vi "Configure Acquisition.vi"(0 "VISA resource name":refnum<visa-resource-name>, 1 "Enable Analog Averaging (Disable)":bool, 2 "Number Of Averages (8)":i32=8, 5 "Acquisition Type (0: Normal)":u16(ring) items=["Normal", "Peak Detect", "High Resolution"], 7 "Sampling Mode  (0: Real Time)":u16(ring) items=["Real Time", "Equivalent Time", "Segment"], 9 "Interpolation (0:No Interpolation)":u16(ring) items=["No Interpolation", "sin(x)/x"], 11 "error in (no error)":errorcluster, 12 "Segment Count (256)":i32=256) -> (4 "VISA resource name out":refnum<visa-resource-name>, 15 "error out":errorcluster)   [LabVIEW 2012, in "Agilent 8000 Series.lvlib"]
doc: "Configures how the oscilloscope acquires data and fills the waveform record."
uses:
  Agilent 8000 Series.lvlib
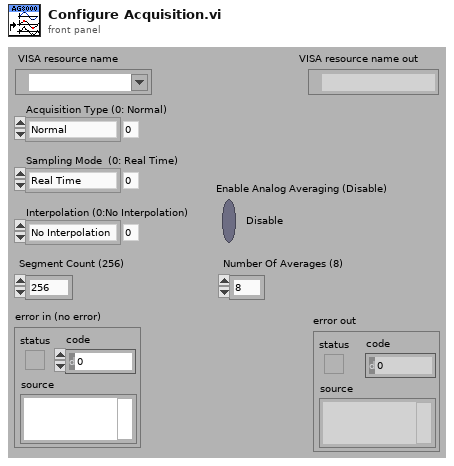
[diagram p1: front panel]
types:
  T1 = enum16{"Real Time", "Peak Detect", "High Resolution"}
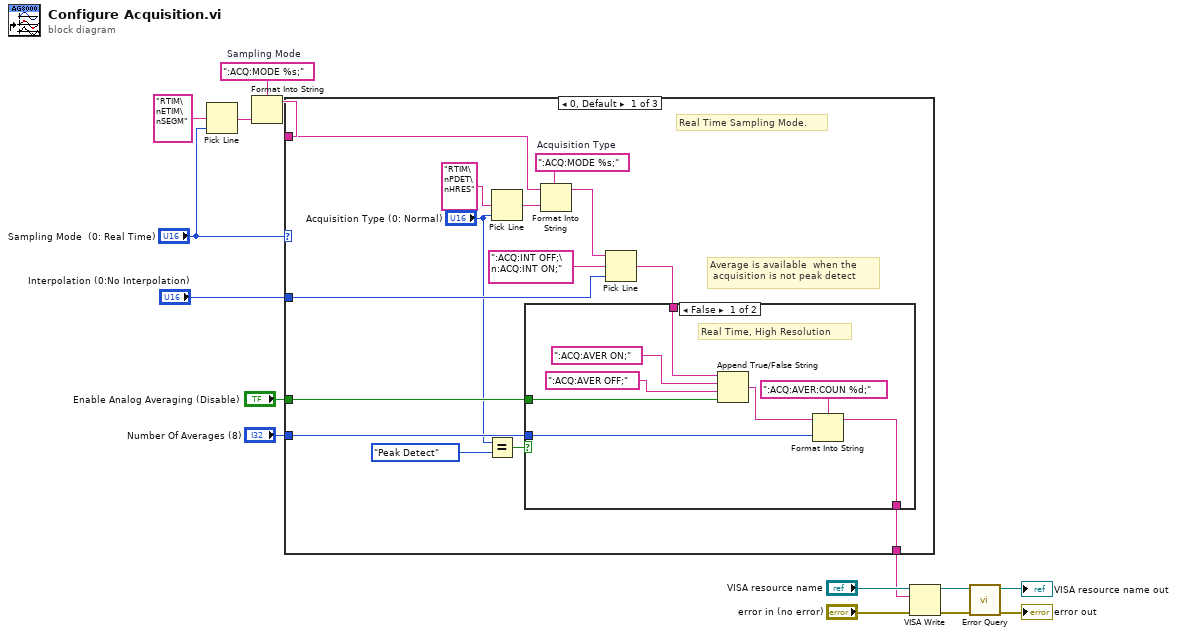
[diagram p0: block diagram]
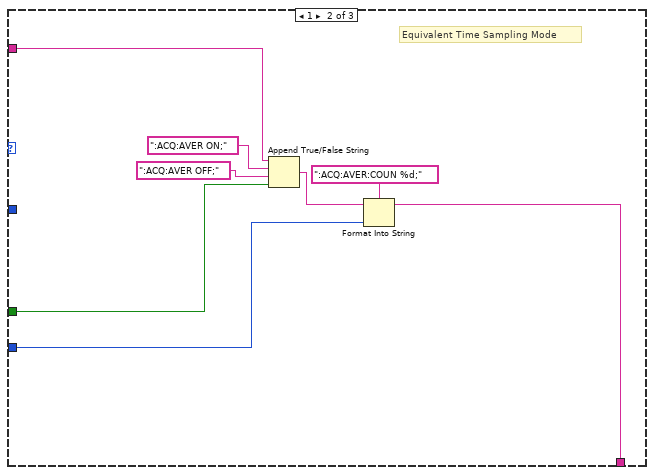
[diagram p3: hidden frame]
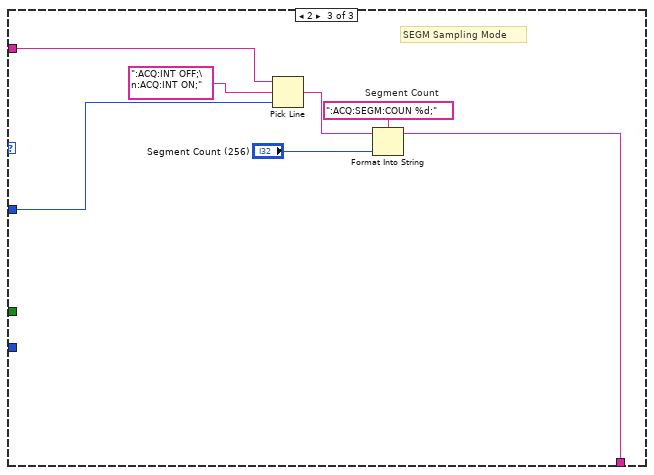
[diagram p4: hidden frame]
diagram:
  w8 = ":ACQ:MODE %s;"  # Sampling Mode
  n1 = Pick Line(multi-line string="RTIM\nETIM\nSEGM", line index="Sampling Mode  (0: Real Time)") -> (output string=w9:string)  [unwired: 1 in]
  n2 = Format Into String(format string=w8, w9) -> (resulting string=w6:string)  [unwired: 2 in, 1 out]
  n3 = case shown="0, Default" "Sampling Mode  (0: Real Time)" {
    tunnel: w6 -> [w16 w45 w52]
    tunnel: "Interpolation (0:No Interpolation)" -> [w28 _ w51]
    tunnel: "Enable Analog Averaging (Disable)" -> [w27 w46 _]
    tunnel: "Number Of Averages (8)" -> [w26 w42 _]
    tunnel: [w24 w39 w47] -> w2
    frame 0, Default {
      w23 = ":ACQ:MODE %s;"  # Acquisition Type
      # "Average is available  when the\n acquisition is not peak detect"
      # "Real Time Sampling Mode."
      n4 = Equal?(x="Acquisition Type (0: Normal)", y=T1."Peak Detect") -> (x = y?=w17:bool)
      n5 = Pick Line(multi-line string="RTIM\nPDET\nHRES", line index="Acquisition Type (0: Normal)") -> (output string=w22:string)  [unwired: 1 in]
      n6 = Format Into String(format string=w23, initial string=w16, w22) -> (resulting string=w20:string)  [unwired: 1 in, 1 out]
      n7 = Pick Line(string ("")=w20, multi-line string=":ACQ:INT OFF;\n:ACQ:INT ON;", line index=w28) -> (output string=w25:string)
      n8 = case shown="False" w17 {
        tunnel: w27 -> [w33 _]
        tunnel: w26 -> [w32 _]
        tunnel: w25 -> [w31 w38]
        tunnel: [w30 w38] -> w24
        frame False {
          # "Real Time, High Resolution"
          n9 = Append True/False String(1:w33, 2:":ACQ:AVER OFF;" ("false string"), 3:":ACQ:AVER ON;" ("true string"), 4:w31) -> (0:w37:string)
          n10 = Format Into String(format string=":ACQ:AVER:COUN %d;", initial string=w37, w32) -> (resulting string=w30:string)  [unwired: 1 in, 1 out]
        }
        frame True {
          # "Peak Detect"
        }
      }
    }
    frame 1 {
      # "Equivalent Time Sampling Mode"
      n11 = Append True/False String(1:w46, 2:":ACQ:AVER OFF;" ("false string"), 3:":ACQ:AVER ON;" ("true string"), 4:w45) -> (0:w40:string)
      n12 = Format Into String(format string=":ACQ:AVER:COUN %d;", initial string=w40, w42) -> (resulting string=w39:string)  [unwired: 1 in, 1 out]
    }
    frame 2 {
      w48 = ":ACQ:SEGM:COUN %d;"  # Segment Count
      # "SEGM Sampling Mode"
      n13 = Pick Line(string ("")=w52, multi-line string=":ACQ:INT OFF;\n:ACQ:INT ON;", line index=w51) -> (output string=w49:string)
      n14 = Format Into String(format string=w48, initial string=w49, "Segment Count (256)") -> (resulting string=w47:string)  [unwired: 1 in, 1 out]
    }
  }
  n15 = VISA Write(VISA resource name="VISA resource name", write buffer=w2, error in (no error)="error in (no error)") -> (VISA resource name out=w14:refnum<visa-resource-name>, error out=w15:errorcluster)  [unwired: 1 out]
  n16 = call "Error Query.vi"("error in (no error)"=w15, "VISA resource name"=w14) -> ("error out"=→"error out":errorcluster, "VISA resource name out"=→"VISA resource name out":refnum<visa-resource-name>)  [unwired: 6 in, 2 out]
